vi "Metadata to listbox.vi"(0 "reference in":refnum<class "XYgraph.lvclass">, 5 "error in (no error)":errorcluster, 8 "Fcurve Metadata ref":refnum<vi>) -> (14 "reference out":refnum<class "XYgraph.lvclass">, 16 "Fcurve Metadata":string[][](table), 19 "error out":errorcluster)   [LabVIEW 2019, in "XYgraph.lvclass"]
doc: "Convert metadata to listbox"
uses:
  XYgraph.lvclass
  Fcurve_class/Loaded Fcurve parameters.ctl
  TDMS_DataHandler_class/PSnex TDMS fcurve property names.ctl
  <vilib>/Utility/miscctls.llb/LVRowAndColumnUnsignedTypeDef.ctl
  <vilib>/Utility/miscctls.llb/LVRowAndColumnTypeDef.ctl
  TDMS_DataHandler_class/TDMS_DataHandler.lvclass
  Fcurve_class/Fcurve.lvclass
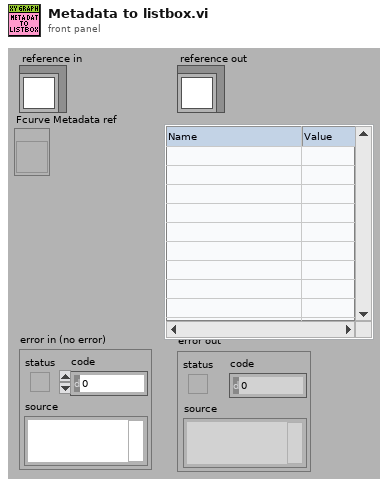
[diagram p1: front panel]
types:
  T1 = typedef "Fcurve.lvclass/Loaded Fcurve parameters.ctl" = T2[]
  T2 = typedef "TDMS_DataHandler.lvclass/PSnex TDMS fcurve property names.ctl" = string
  T3 = typedef "LVRowAndColumnUnsignedTypeDef.ctl" = cluster{"Row":u32, "Column":u32}
  T4 = typedef "LVRowAndColumnTypeDef.ctl" = cluster{"Row":i32, "Column":i32}
  T5 = typedef "XYgraph.lvclass/ObjectAttributes.ctl" = cluster{"FPref":T6, "MyAttribute":dbl, "X multiplier":dbl, "Y multiplier":dbl, "X Scale name":string, "Y Scale name":string, "Fcurve metadata":T7, "Fcurve":refnum<class "Fcurve.lvclass">}
  T6 = typedef "XYgraph.lvclass/XY graph ref.ctl" = refnum<vi>
  T7 = typedef "Fcurve.lvclass/Metadata.ctl" = cluster{"dt (us)":dbl, "Dec Factor":dbl, "Z piezo Sensitivity (nm/V)":dbl, "K (N/m)":dbl, "Sp (V)":dbl, "Contact (ms)":dbl, "Zpos contact":dbl, "Vel_app (nm/s)":dbl, "Vel_ret (nm/s)":dbl, "deltaV (nm)":dbl, "Def_V0 (v)":dbl, "Piezo gain":dbl, "invOLS (nm/V)":dbl}
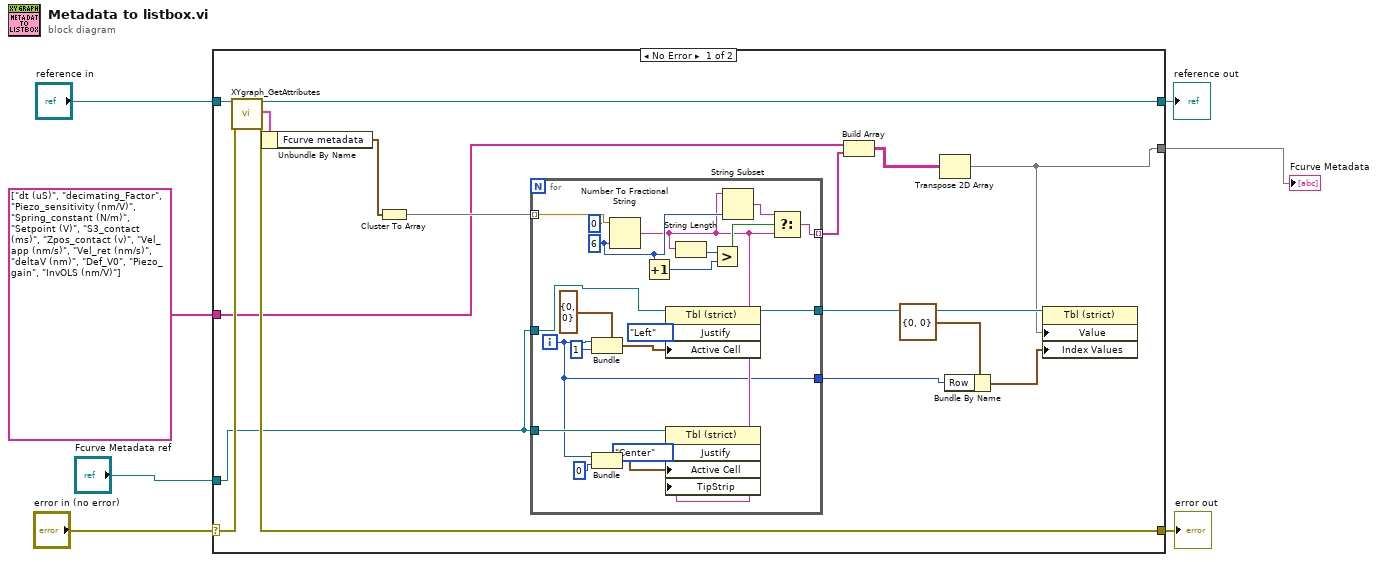
[diagram p0: block diagram]
diagram:
  n1 = case shown="No Error" "error in (no error)" {
    selector: "error in (no error)" -> [w23 w45]
    tunnel: [w22 w45] -> w6
    tunnel: [w21 w44] -> w4
    tunnel: "reference in" -> [w19 w44]
    tunnel: T1 ["dt (uS)", "decimating_Factor", "Piezo_sensitivity (nm/V)", "Spring_constant (N/m)", "Setpoint (V)", "S3_contact (ms)", "Zpos_contact (v)", "Vel_app (nm/s)", "Vel_ret (nm/s)", "deltaV (nm)", "Def_V0", "Piezo_gain", "InvOLS (nm/V)"] ("Loaded Fcurve parameters") -> [w17 _]
    tunnel: [w11 _] -> w2
    tunnel: "Fcurve Metadata ref" -> [w13 _]
    frame No Error {
      n2 = call "XYgraph_GetAttributes.vi"("reference in"=w19, "error in (no error)"=w23) -> ("reference out"=w21:refnum<class "XYgraph.lvclass">, "attributes"=w20:T5, "error out"=w22:errorcluster)  [unwired: 14 in, 1 out]
      n3 = Unbundle By Name(w20) -> ("Fcurve metadata"=w16:T7)
      n4 = Cluster To Array(cluster=w16) -> (array=w18:dbl[])
      n5 = for {
        tunnel: w18 -> [w43] mode=indexing
        tunnel: [w32] -> w15 mode=indexing
        tunnel: w13 -> [w27]
        tunnel: w13 -> [w26]
        tunnel: [w25] -> w12
        tunnel: [w24] -> w8
        i -> [w24]
        w30 = i16 6 ("precision (6)")
        n6 = Bundle(cluster=T4 {"Row"=0, "Column"=0} ("Active Cell:Active Cell"), "Row"=w24, "Column"=1) -> (w38:T4)
        n7 = Bundle(w24, "Column"=0) -> (w36:cluster{i32, "Column":i32})  [unwired: 1 in]
        n8 = Number To Fractional String(number=w43, width (-)=i16 0, precision (6)=w30) -> (F-format string=w28:string)  [unwired: 1 in]
        n9 = Increment(x=w30) -> (x+1=w29:i16)
        n10 = property on="Property Node" class="Tbl (strict)"(reference=w26, "Justify"=enum16{"Left", "Center", "Right"}."Left" ("Active Cell:Cell Justification"), "Active Cell"=w38) -> (reference out=w25:refnum<vi>)  [unwired: 1 in, 1 out]
        n11 = property on="Property Node" class="Tbl (strict)"(reference=w27, "Justify"=enum16{"Left", "Center", "Right"}."Center" ("Active Cell:Cell Justification"), "Active Cell"=w36, "TipStrip"=w28) -> ()  [unwired: 1 in, 2 out]
        n12 = String Length(string=w28) -> (length=w34:i32)
        n13 = Greater?(x=w34, y=w29) -> (0:w33:bool)
        n14 = String Subset(string=w28, length (rest)=w30) -> (substring=w31:string)  [unwired: 1 in]
        n15 = Select(t=w31, s=w33, f=w28) -> (s? t:f=w32:string)
      }
      n16 = Build Array(w17, w15) -> (w14:T2[][])
      n17 = Transpose 2D Array(2D array=w14) -> (transposed array=w11:T2[][])
      n18 = Bundle By Name(cluster=T3 {"Row"=0, "Column"=0} ("Index Values"), "Row"=w8) -> (w9:T3)
      n19 = property on="Property Node" class="Tbl (strict)"(reference=w12, "Value"=w11, "Index Values"=w9) -> ()  [unwired: 1 in, 2 out]
    }
    frame Error {
    }
  }
  "error out" <- w6
  "reference out" <- w4
  "Fcurve Metadata" <- w2
